vi "BELLA-VIremote-Master.vi"() -> ()   [LabVIEW 2011]
uses:
  VIremote.llb/VIremoteFunction.ctl
  VIremote.llb/VIremoteNavigationBar.ctl
  VIremote.llb/VIremoteStatus.ctl
panel:
  in  "Use emulation":bool
  in  "Make Palette":bool
  in  "Select demo ring":i16(ring) caption="Select Demo" items=["Bella_M1Cam_GUI-viremote.vi", "Bella_M2Cam_GUI-viremote.vi", "Bella_M4Cam_GUI-viremote.vi", "Bella_M5Cam_GUI-viremote.vi", "-", "QUIT"]
  in  "ggg":bool
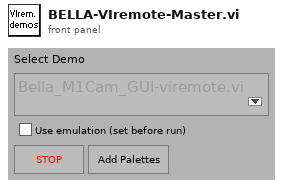
[diagram p1: front panel]
types:
  T1 = typedef "VIremoteNavigationBar.ctl" = enum16{"Show Bar", "Hide Bar", "Clear History", "Set Bar Tint Color", "Set Bar Title", "Set Bar Prompt", "Show Back Button", "Hide Back Button", "Set Back Button Text", "Add Right Button", "Add Left Button", "Remove Button"}
  T2 = typedef "VIremoteFunction.ctl" = enum16{"Do nothing", "Stop controller", "Close this connection", "Show info panel", "Set VI to control", "Set Accelerometer freq (Hz)", "Show Alert message", "Start Sound Input", "Stop Sound Input", "Set Volume (0-100)", "Set sound output Speaker", "Set sound output Receiver", "Play Sound", "Repeat Sound", "Stop Sound", "Pause Sound", "Resume Sound", "Set panel width of caller (320 or 480)", "Set Panel Size to Portrait", "Set Panel Size to Landscape", "Set Panel Size as Current Orientation", "Allow all UI Orientations", "Send user notification", "Disable Scrolling", "Normal Scrolling", "Page Scrolling", "Set Scroll Offset", "Page Indicator Position"}
  T3 = typedef "VIremoteStatus.ctl" = enum16{"Connected BOOL", "Number of connections DBL", "VIremoteController ver.", "VIremote ver. DBL", "Screen width DBL", "Screen height DBL", "Current navigation bar height DBL", "Current UI orientation", "Background supported BOOL", "Background state BOOL", "Device UI idiom (0=phone,1=iPad) DBL", "Device name", "Device unique id", "Device system ver.", "Device model", "Device HW model"}
  T4 = typedef "VIremoteInit.ctl" = cluster{"port (2055)":u16, "Use mouse emulation (T)":bool, "Use keyboard emulation (T)":bool, "Allow multiple connections (F)":bool, "Debug mode/error dialog (F)":bool, "Temporary directory (default)":path, "Mouse emulation VI path":path, "Keyboard emulation VI path":path, "Enable VI Select button(T)":bool, "Enable auto scroll(T)":bool}
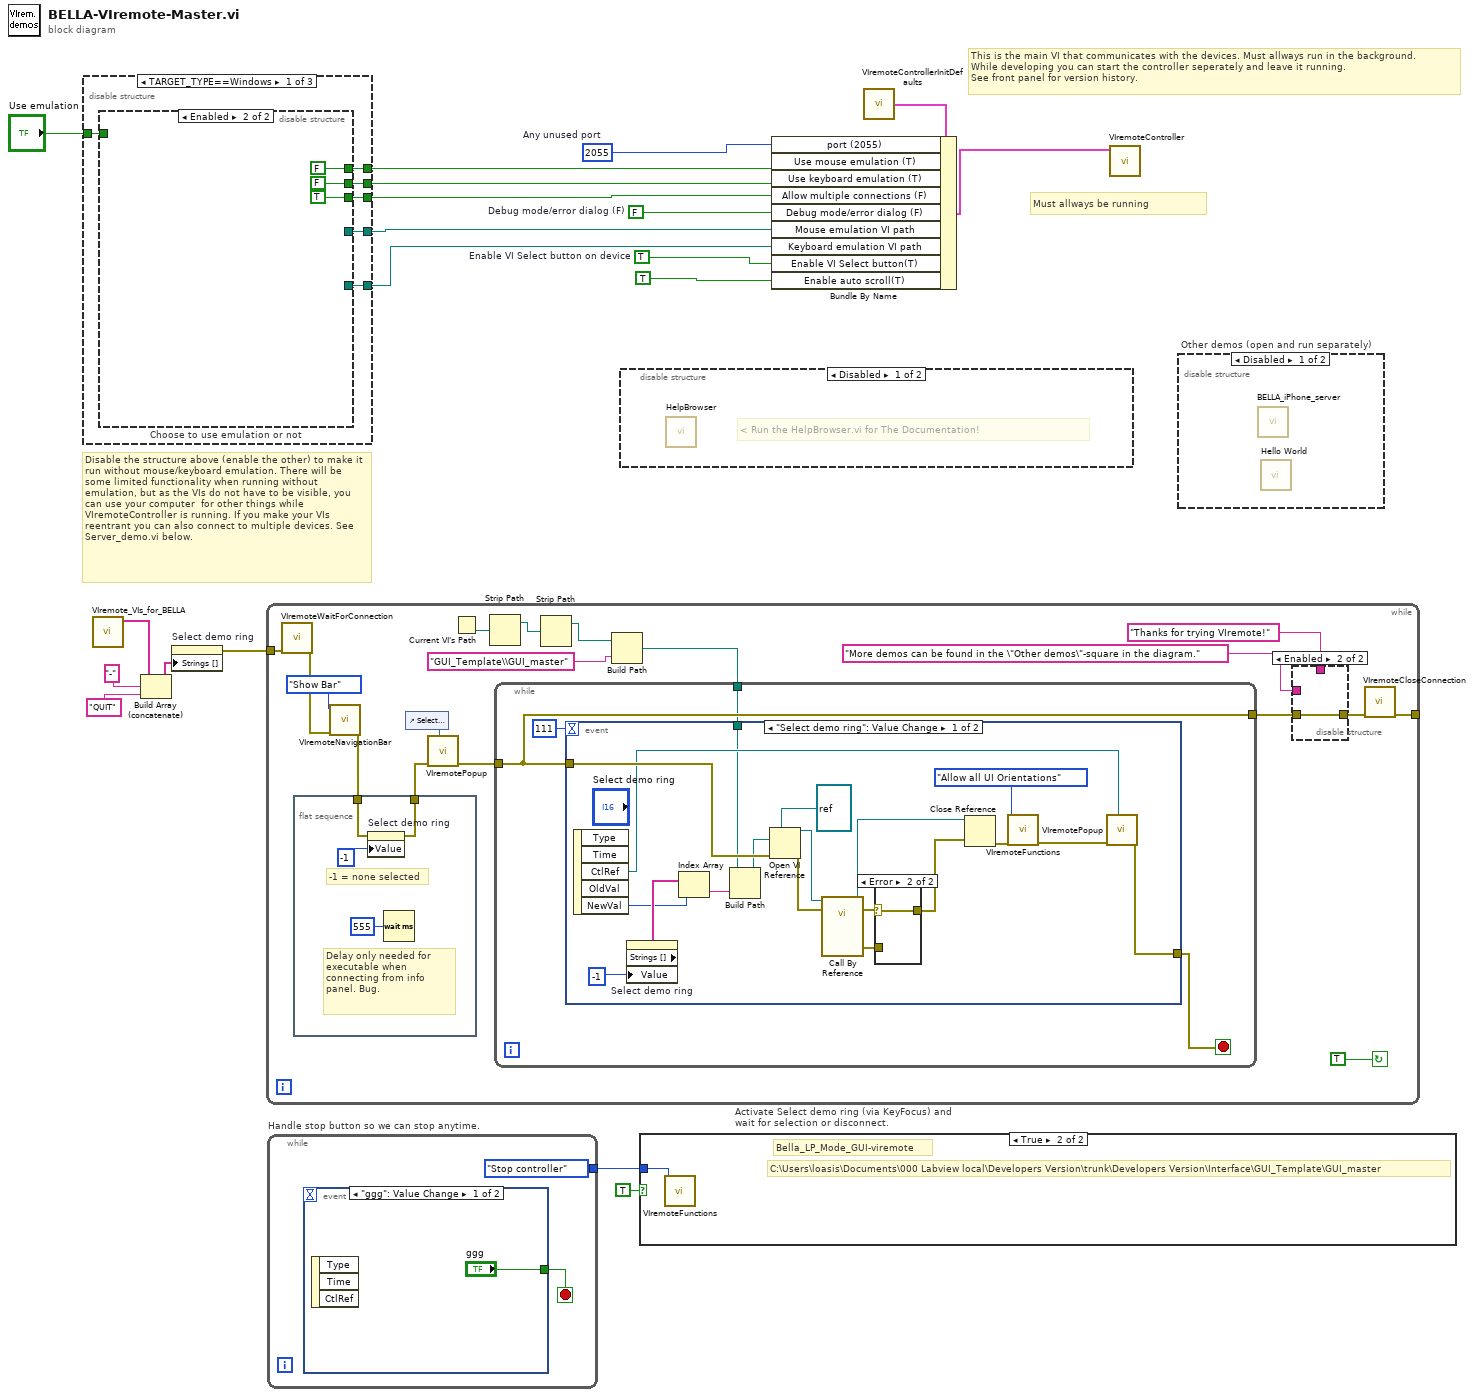
[diagram p0: block diagram]
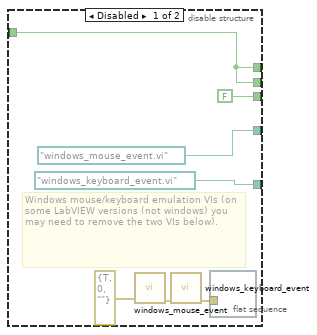
[diagram p4: hidden frame]
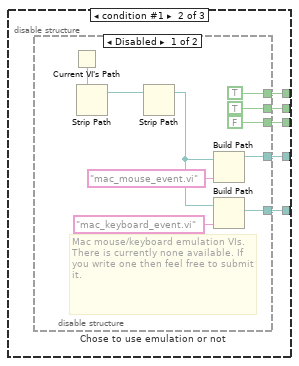
[diagram p5: hidden frame]
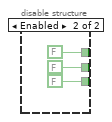
[diagram p6: hidden frame]
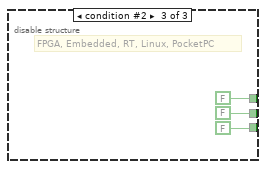
[diagram p7: hidden frame]
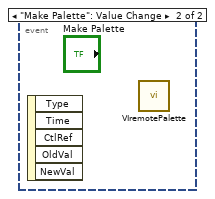
[diagram p8: hidden frame]
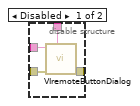
[diagram p9: hidden frame]
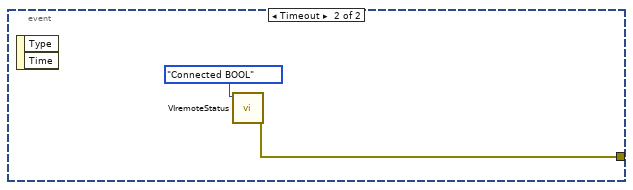
[diagram p11: hidden frame]
diagram:
  w10 = TRUE  # Enable VI Select button on device
  w18 = FALSE  # Debug mode/error dialog (F)
  w19 = u16 2055  # Any unused port
  # "< Run the HelpBrowser.vi for The Documentation!"
  # "Disable the structure above (enable the other) to make it run without mouse/keyboard emulation. There will be some limited functionality when running without emulation, but as the VIs do not have to be visible, you can use your computer  for other things while VIremoteController is running. If you make your VIs reentrant you can also connect to multiple devices. See Server_demo.vi below."
  # "Must allways be running"
  # "This is the main VI that communicates with the devices. Must allways run in the background.\nWhile developing you can start the controller seperately and leave it running.\nSee front panel for version history."
  n1 = disable-structure shown="TARGET_TYPE==Windows" {
    disable-tunnel: [w25 w40 _] -> w16
    disable-tunnel: [w24 w39 _] -> w15
    disable-tunnel: [w23 w38 FALSE ("Use mouse emulation (T)")] -> w13
    disable-tunnel: [w22 w37 FALSE ("Use keyboard emulation (T)")] -> w12
    disable-tunnel: [w21 w36 FALSE ("Allow multiple connections (F)")] -> w11
    disable-tunnel: "Use emulation" -> [w20 _ _]
    frame condition #0 (active) {
      n2 = disable-structure "Choose to use emulation or not" shown="Enabled" {
        disable-tunnel: [path "windows_mouse_event.vi" ("name or relative path") _] -> w25
        disable-tunnel: [path "windows_keyboard_event.vi" ("name or relative path") _] -> w24
        disable-tunnel: [w28 FALSE ("Use mouse emulation (T)")] -> w23
        disable-tunnel: [w28 FALSE ("Use keyboard emulation (T)")] -> w22
        disable-tunnel: [FALSE ("Allow multiple connections (F)") TRUE ("Allow multiple connections (F)")] -> w21
        disable-tunnel: w20 -> [w28 _]
        frame Disabled {
          # "Windows mouse/keyboard emulation VIs (on some LabVIEW versions (not windows) you may need to remove the two VIs below)."
          n3 = call "windows_mouse_event.vi"("error in (no error)"=errorcluster {"status"=TRUE, "code"=0, "source"=""}) -> ("error out"=w30:errorcluster)  [unwired: 4 in, 6 out]
          n4 = call "windows_keyboard_event.vi"("error in (no error)"=w30) -> ("error out"=w29:errorcluster)  [unwired: 1 in, 9 out]
          n5 = flat-sequence {
            tunnel: w29 -> [_]
            frame #0 {
            }
          }
        }
        frame Enabled {
        }
      }
    }
    frame condition #1 {
      n6 = disable-structure "Chose to use emulation or not" shown="Disabled" {
        disable-tunnel: [w45 _] -> w40
        disable-tunnel: [w44 _] -> w39
        disable-tunnel: [TRUE ("Use mouse emulation (T)") FALSE ("Use mouse emulation (T)")] -> w38
        disable-tunnel: [TRUE ("Use keyboard emulation (T)") FALSE ("Use keyboard emulation (T)")] -> w37
        disable-tunnel: [FALSE ("Allow multiple connections (F)") FALSE ("Allow multiple connections (F)")] -> w36
        frame Disabled {
          # "Mac mouse/keyboard emulation VIs. There is currently none available. If you write one then feel free to submit it."
          n7 = Current VI's Path() -> (path=w42:path)
          n8 = Strip Path(path=w42) -> (stripped path=w43:path)  [unwired: 1 out]
          n9 = Strip Path(path=w43) -> (stripped path=w41:path)  [unwired: 1 out]
          n10 = Build Path(base path=w41, name or relative path="mac_mouse_event.vi") -> (appended path=w45:path)
          n11 = Build Path(base path=w41, name or relative path="mac_keyboard_event.vi") -> (appended path=w44:path)
        }
        frame Enabled {
        }
      }
    }
    frame condition #2 {
      # "FPGA, Embedded, RT, Linux, PocketPC"
    }
  }
  n12 = call "VIremote_VIs_for_BELLA.vi"() -> ("Strings []"=w2:string[])  [unwired: 10 in, 1 out]
  n13 = Build Array (concatenate)(w2, "-", "QUIT") -> (w8:string[])
  n14 = property on="Select demo ring" class="Ring (strict)"("Strings []"=w8) -> (error out=w9:errorcluster)  [unwired: 2 in, 1 out]
  n15 = while "Activate Select demo ring (via KeyFocus) and wait for selection or disconnect." {
    tunnel: [w73] -> _
    tunnel: w9 -> [w69]
    stop <- TRUE continue-if-true
    n16 = call "VIremoteWaitForConnection.vi"("error in (no error)"=w69) -> ("error out"=w62:errorcluster)  [unwired: 10 out]
    n17 = flat-sequence {
      tunnel: [w82] -> w67
      tunnel: w63 -> [w81]
      frame #0 {
        # "Delay only needed for executable when connecting from info panel. Bug."
        # "-1 = none selected"
        n18 = property on="Select demo ring" class="Ring (strict)"(error in=w81, "Value"=-1) -> (error out=w82:errorcluster)  [unwired: 1 in, 1 out]
        n19 = Wait (ms)(milliseconds to wait=u32 555) -> ()  [unwired: 1 out]
      }
    }
    n20 = call "VIremoteNavigationBar.vi"("error in (no error)"=w62, "Func"=VIremoteNavigationBar."Show Bar") -> ("error out"=w63:errorcluster)  [unwired: 3 in, 6 out]
    n21 = control-ref of="Select demo ring"() -> (w65:refnum<vi>)
    n22 = call "VIremotePopup.vi"("Control Refnum"=w65, "error in (no error)"=w67) -> ("error out"=w64:errorcluster)  [unwired: 1 in, 8 out]
    n23 = Current VI's Path() -> (path=w61:path)
    n24 = Strip Path(path=w61) -> (stripped path=w60:path)  [unwired: 1 out]
    n25 = Strip Path(path=w60) -> (stripped path=w59:path)  [unwired: 1 out]
    n26 = Build Path(base path=w59, name or relative path="GUI_Template\\GUI_master") -> (appended path=w57:path)
    n27 = while {
      tunnel: w64 -> [w86]
      tunnel: [w86] -> w68
      tunnel: w57 -> [w85]
      stop <- w84 stop-if-true
      n28 = event shown="[0] \"Select demo ring\": Value Change" {
        selector: _ -> [_ _]
        dyn-events: _ -> [_ _]
        timeout: 111 -> [_ _]
        tunnel: [w92 w109] -> w84
        tunnel: w86 -> [w97 _]
        tunnel: w85 -> [w88 _]
        event "Select demo ring": Value Change {
          n29 = event-data() -> ("CtlRef"=w93:refnum<vi>, "NewVal"=w105:i16)  [unwired: 4 out]
          n30 = property on="Select demo ring" class="Ring (strict)"("Value"=-1) -> ("Strings []"=w106:string[])  [unwired: 2 in, 2 out]
          n31 = Index Array(array=w106, index=w105) -> (element=w90:string)
          n32 = Build Path(base path=w88, name or relative path=w90) -> (appended path=w89:path)
          n33 = Open VI Reference(type specifier VI Refnum (for type only)=refnum<vi> refnum, vi path=w89, error in (no error)=w97) -> (vi reference=w104:refnum<vi>, error out=w101:errorcluster)  [unwired: 3 out]
          n34 = call-by-ref "?"(reference=w104, error in=w101) -> (reference out=w102:refnum<vi>, error out=w100:errorcluster, 0:"error out"=w99:errorcluster)  [unwired: 11 in]
          n35 = case shown="Error" w100 {
            selector: w100 -> [_ w108]
            tunnel: w99 -> [w107 _]
            tunnel: [w107 w108] -> w98
            frame No Error {
            }
            frame Error {
            }
          }
          n36 = Close Reference(reference=w102, error in (no error)=w98) -> (error out=w95:errorcluster)
          n37 = call "VIremoteFunctions.vi"("error in (no error)"=w95, "Function"=VIremoteFunction."Allow all UI Orientations") -> ("error out"=w91:errorcluster)  [unwired: 4 in, 5 out]
          n38 = call "VIremotePopup.vi"("Control Refnum"=w93, "error in (no error)"=w91) -> ("error out"=w92:errorcluster)  [unwired: 9 out]
        }
        event Timeout {
          n39 = event-data() -> ()  [unwired: 3 out]
          n40 = call "VIremoteStatus.vi"("Status item"=VIremoteStatus."Connected BOOL") -> ("error out"=w109:errorcluster)  [unwired: 2 in, 8 out]
        }
      }
    }
    n41 = disable-structure shown="Enabled" {
      disable-tunnel: "More demos can be found in the \"Other demos\"-square in the diagram." ("message") -> [w78 _]
      disable-tunnel: [w77 w79] -> w71
      disable-tunnel: "Thanks for trying VIremote!" ("message") -> [w76 _]
      disable-tunnel: w68 -> [w75 w79]
      frame Disabled {
        n42 = call "VIremoteButtonDialog.vi"("Window Title (\"\")"=w76, "error in (no error)"=w75, "message"=w78) -> ("error out"=w77:errorcluster)  [unwired: 1 in, 7 out]
      }
      frame Enabled {
      }
    }
    n43 = call "VIremoteCloseConnection.vi"("error in (no error)"=w71) -> ("error out"=w73:errorcluster)  [unwired: 1 in, 9 out]
  }
  n44 = while "Handle stop button so we can stop anytime." {
    tunnel: [VIremoteFunction."Stop controller" ("Function")] -> w14
    stop <- w112 stop-if-true
    n45 = event shown="[0] \"ggg\": Value Change" {
      selector: _ -> [_ _]
      dyn-events: _ -> [_ _]
      timeout: _ -> [_ _]
      tunnel: ["ggg" _] -> w112
      event "ggg": Value Change {
        n46 = event-data() -> ()  [unwired: 4 out]
      }
      event "Make Palette": Value Change {
        n47 = event-data() -> ()  [unwired: 6 out]
        n48 = call "VIremotePalette.vi"() -> ()  [unwired: 1 out]
      }
    }
  }
  n49 = disable-structure shown="Disabled" {
    frame Disabled {
      n50 = call "HelpBrowser.vi"() -> ()  [unwired: 1 in]
    }
    frame Enabled {
    }
  }
  n51 = case shown="True" TRUE {
    tunnel: w14 -> [_ w114]
    frame False {
    }
    frame True {
      # "Bella_LP_Mode_GUI-viremote"
      # "C:\\Users\\loasis\\Documents\\000 Labview local\\Developers Version\\trunk\\Developers Version\\Interface\\GUI_Template\\GUI_master"
      n52 = call "VIremoteFunctions.vi"("Function"=w114) -> ()  [unwired: 5 in, 6 out]
    }
  }
  n53 = call "VIremoteControllerInitDefaults.vi"() -> ("Init defaults"=w4:T4)
  n54 = Bundle By Name(cluster=w4, "port (2055)"=w19, "Use mouse emulation (T)"=w13, "Use keyboard emulation (T)"=w12, "Allow multiple connections (F)"=w11, "Debug mode/error dialog (F)"=w18, "Mouse emulation VI path"=w16, "Keyboard emulation VI path"=w15, "Enable VI Select button(T)"=w10, "Enable auto scroll(T)"=TRUE) -> (w17:T4)
  n55 = call "VIremoteController.vi"("Init (can't be changed while running)"=w17) -> ()  [unwired: 11 out]
  n56 = disable-structure "Other demos (open and run separately)" shown="Disabled" {
    frame Disabled {
      n57 = call "BELLA_iPhone_server.vi"() -> ()  [unwired: 1 out]
      n58 = call "Hello World.vi"() -> ()  [unwired: 1 in]
    }
    frame Enabled {
    }
  }
